vi "SVT Get Octave Value (1 Ch).vi"(0 "octave spectrum":T5 {"band power" format="%.2f"; "nominal frequencies [Hz]" format="%.2f"}, 5 "frequency [Hz]":dbl=1000.0 format="%.2f", 9 "octave info":T1={"standard"=enum."ANSI S1.11", "bandwidth"=enum."1 octave", "low band"=0, "high band"=0, "weighting filter"=0, "dB reference"=0.0, "dB On"=FALSE, "unit label"="", "channel name"="", "description"="", "engineering units"=1, "custom label"="", "spectrum type"=enum."magnitude", "spectral density"=FALSE, "filters settled"=FALSE} {"engineering units" items=["custom..."=0, "V"=1, "A"=21, "C"=30, "pC"=31, "s"=32, "-"=29, "Pa"=2, "N"=20, "g"=3, "m/s^2"=4, "m/s"=5, "m"=6, "mm/s"=12, "mm"=13, "micron/s"=14, "micron"=15, "in/s^2"=7, "in/s"=8, "in"=9, "mil/s"=10, "mil"=11, "rad/s^2"=16, "rad/s"=17, "rad"=18, "deg/s^2"=26, "deg/s"=27, "deg"=28, "RPM"=22, "cycle/s^2"=23, "Hz"=24, "cycle"=25, "strain"=19]; "dB reference" format="%.2e"; "weighting filter" items=["Linear", "A-weighting", "B-weighting", "C-weighting", "ITU-R 468-4", "Dolby", "CCITT", "C-message", "Wb", "Wc", "Wd", "We", "Wf", "Wh", "Wj", "Wk", "Wm", "AES17 20 kHz lowpass", "AES17 40 kHz lowpass", "AES17 20 kHz highpass", "AES17 40 kHz highpass"]}, 11 "error in (no error)":errorcluster) -> (4 "band power value":dbl=nan format="%.2p", 6 "unit label":string, 8 "actual nominal frequency [Hz]":dbl=nan format="%.2f", 15 "error out":errorcluster)   [LabVIEW 2017, in "SoundVib_Octave_2014 standard.lvlib"]
doc: "Extracts the band power value of the <B>octave spectrum</B> at the specified input frequency. Finds the octave band that corresponds to the input frequency if the input frequency does not exactly coincide with a nominal frequency. Wire data to the <B>octave spectrum</B> input to determine the polymorphic instance to use or manually select the instance."
uses:
  <vilib>/addons/Sound and Vibration/svt_Octave/SoundVib_Octave_2014 standard.lvlib
  <vilib>/addons/_NISVFA/_Shared subVIs/Controls/svc_Octave Info.ctl
  <vilib>/addons/_NISVFA/_Shared subVIs/Controls/svc_Octave Standard.ctl
  <vilib>/addons/_NISVFA/_Shared subVIs/Controls/svc_Weighting Filter Text Ring.ctl
  <vilib>/addons/_NISVFA/_Shared subVIs/Controls/svc_Engineering Units Text Ring.ctl
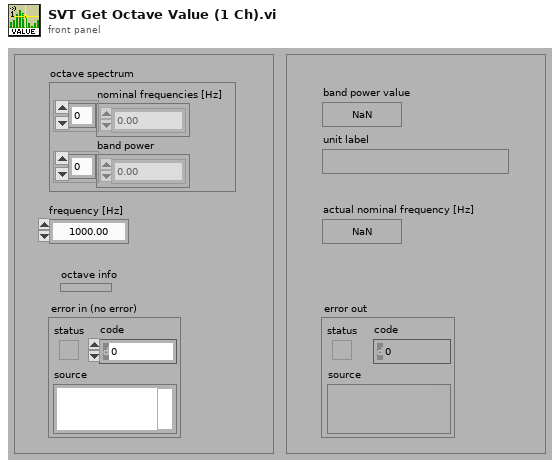
[diagram p1: front panel]
types:
  T1 = typedef "svc_Octave Info.ctl" = cluster{"standard":T2, "bandwidth":enum16{"1 octave", "1/3 octave", "1/6 octave", "1/12 octave", "1/24 octave"}, "low band":i32, "high band":i32, "weighting filter":T3, "dB reference":dbl, "dB On":bool, "unit label":string, "channel name":string, "description":string, "engineering units":T4, "custom label":string, "spectrum type":enum16{"power", "magnitude"}, "spectral density":bool, "filters settled":bool}
  T2 = typedef "svc_Octave Standard.ctl" = enum16{"ANSI S1.11", "IEC 61260"}
  T3 = typedef "svc_Weighting Filter Text Ring.ctl" = u16
  T4 = typedef "svc_Engineering Units Text Ring.ctl" = u16
  T5 = cluster{"nominal frequencies [Hz]":dbl[], "band power":dbl[]}
  T6 = cluster{"f low":dbl, "f high":dbl, "midband":dbl}[]
  T7 = cluster{"f low":dbl, "f high":dbl, "midband":dbl}
  T8 = enum16{"1 octave", "1/3 octave", "1/6 octave", "1/12 octave", "1/24 octave"}
  T9 = cluster{"frequency [Hz]":dbl, "frequency [Hz]":dbl}
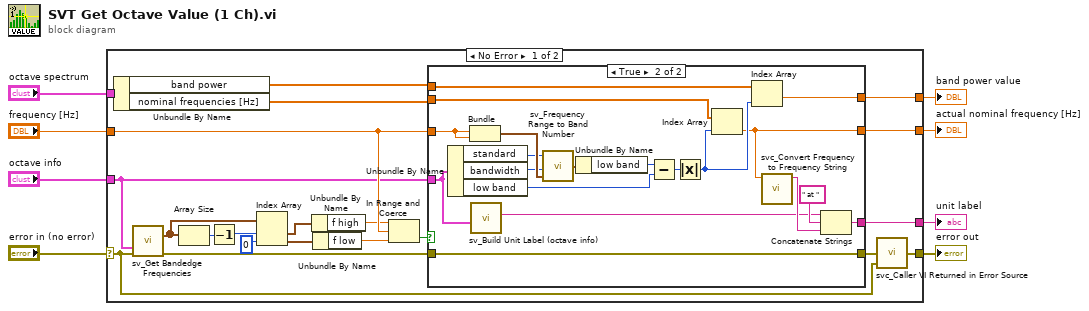
[diagram p0: block diagram]
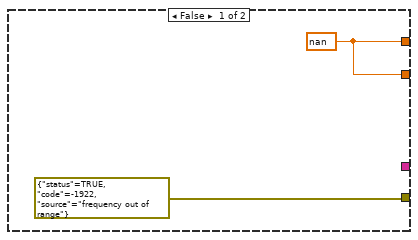
[diagram p2: hidden frame]
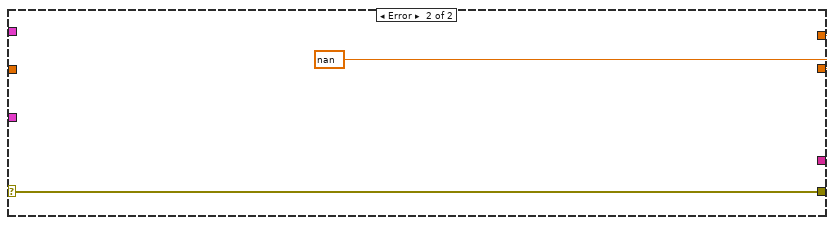
[diagram p3: hidden frame]
diagram:
  n1 = case shown="No Error" "error in (no error)" {
    selector: "error in (no error)" -> [w13 w52]
    tunnel: [w20 w52] -> w8
    tunnel: "octave spectrum" -> [w29 _]
    tunnel: [w28 _] -> w6
    tunnel: "octave info" -> [w14 _]
    tunnel: "frequency [Hz]" -> [w24 _]
    tunnel: [w27 w51] -> w3
    tunnel: [w26 w51] -> w2
    frame No Error {
      n2 = Unbundle By Name(w29) -> ("band power"=w23:dbl[], "nominal frequencies [Hz]"=w22:dbl[])
      n3 = call <vilib>:"sv_Get Bandedge Frequencies.vi"("octave info"=w14, "error in (no error)"=w13) -> ("bandedge frequencies [Hz]"=w16:T6, "error out"=w12:errorcluster)  [unwired: 12 in]
      n4 = Array Size(array=w16) -> (size(s)=w19:i32)
      n5 = Decrement(x=w19) -> (x-1=w18:i32)
      n6 = Index Array(array=w16, index #1=w18, index #2=0 ("index")) -> (element #1=w15:T7, element #2=w11:T7)
      n7 = Unbundle By Name(w15) -> ("f high"=w10:dbl)
      n8 = Unbundle By Name(w11) -> ("f low"=w9:dbl)
      n9 = In Range and Coerce(upper limit=w10, x=w24, lower limit=w9) -> (In Range?=w25:bool)  [unwired: 1 out]
      n10 = case shown="True" w25 {
        tunnel: w14 -> [_ w33]
        tunnel: w12 -> [_ w46]
        tunnel: [errorcluster {"status"=TRUE, "code"=-1922, "source"="frequency out of range"} ("error out") w46] -> w21
        tunnel: w22 -> [_ w38]
        tunnel: [_ w50] -> w28
        tunnel: [w30 w34] -> w27
        tunnel: [w30 w39] -> w26
        tunnel: w24 -> [_ w47]
        tunnel: w23 -> [_ w40]
        frame False {
          w30 = nan ("frequency [Hz]")
        }
        frame True {
          n11 = Unbundle By Name(w33) -> ("standard"=w43:T2, "bandwidth"=w42:T8, "low band"=w35:i32)
          n12 = Bundle("frequency [Hz]"=w47, "frequency [Hz]"=w47) -> (w45:T9)  [unwired: 1 in]
          n13 = call <vilib>:"sv_Build Unit Label (octave info).vi"("octave info"=w33) -> ("unit label"=w32:string)  [unwired: 8 in, 2 out]
          n14 = call <vilib>:"sv_Frequency Range to Band Number.vi"("frequency range [Hz]"=w45, "bandwidth"=w42, "standard"=w43) -> ("band number"=w44:cluster{"low band":i32, "high band":i32})
          n15 = Unbundle By Name(w44) -> ("low band"=w36:i32)
          n16 = Subtract(x=w36, y=w35) -> (x-y=w41:i32)
          n17 = Absolute Value(x=w41) -> (abs(x)=w37:i32)
          n18 = Index Array(array=w38, index=w37) -> (element=w34:dbl)
          n19 = Index Array(array=w40, index=w37) -> (element=w39:dbl)
          n20 = call <vilib>:"svc_Convert Frequency to Frequency String.vi"("frequency [Hz]"=w34) -> ("frequency string"=w48:string)  [unwired: 10 in]
          n21 = Concatenate Strings(w32, " at " ("string"), w48) -> (w50:string)
        }
      }
      n22 = call <vilib>:"svc_Caller VI Returned in Error Source.vi"("warning input to caller"=w13, "error in (no error)"=w21) -> ("error out"=w20:errorcluster)  [unwired: 3 in]
    }
    frame Error {
      w51 = nan ("frequency [Hz]")
    }
  }
  "error out" <- w8
  "unit label" <- w6
  "actual nominal frequency [Hz]" <- w3
  "band power value" <- w2
